vi "generateCommand.vi"(1 "IP":string, 2 "CommandProtoType":string) -> (0 "Command":string)   [LabVIEW 2010]
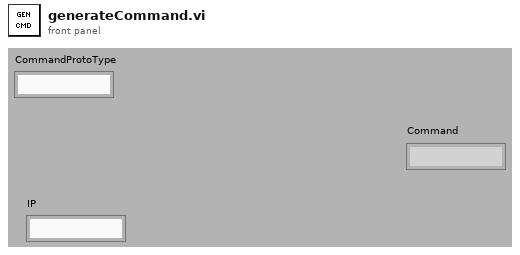
[diagram p1: front panel]
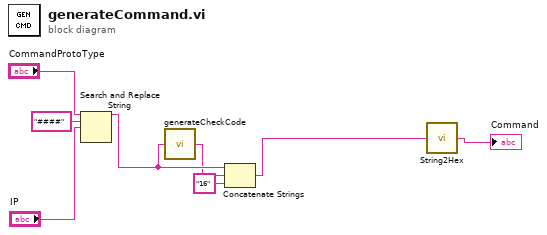
[diagram p0: block diagram]
diagram:
  n1 = Search and Replace String(input string="CommandProtoType", search string="####", replace string="IP") -> (result string=w4:string)  [unwired: 5 in, 3 out]
  n2 = call "generateCheckCode.vi"("Data"=w4) -> ("CheckCode"=w3:string)
  n3 = Concatenate Strings(w4, w3, "16" ("string")) -> (w1:string)
  n4 = call "String2Hex.vi"("value"=w1) -> ("String"=→"Command":string)
